vi "Open_File_for_write_check.vi"(8 "advisory dialog? (display:T)":bool=TRUE, 9 "append to file? (new file:F)":bool, 11 "file path":path) -> (0 "error out":errorcluster, 3 "refnum":refnum<file>)   [LabVIEW 2021]
doc: "Opens an existing file, creates a new file, or replaces an existing file, programmatically or interactively using dialog. You can optionally specify a dialog prompt, default file name, start path, or filter pattern, and you can specify open and deny modes when opening a file, plus group and permission when creating a new file. Use this VI with the intermediate Write File+ or Read File+ VIs described below.\n\nfile path is the path name of the file. If file path is empty (default value) or is Not A Path, the VI displays a File dialog box from which you can select a file. Error 43 occurs if the user cancels the dialog. \n\nfunction is the operation to perform:\n\n 0 (open) opens an existing file. Error 7 occurs if the file cannot be found.\n \n 1 (open or create) opens an existing file or creates a new file if one does not exist.\n\n 2 (create or replace) creates a new file or replaces a file if it exists and you give permission. Replacement is done by opening the file and setting EOF to 0. Error 43 occurs if the user elects to disallow the replacement using dialog. \n\n 3 (create) creates a new file. Error 8 occurs if the file already exists.\n\nadvisory dialog? Set TRUE (default) if you want a dialog if function=0 and the file does not exist, or if function=2 or 3 and the file exists.\n\nprompt is the message that appears below the list of files and directories in the file dialog.\n\ndefault name is the initial file name that appears in the selection box of the file dialog.\n\nstart path is the path name to the initially displayed directory in a file dialog. The default value is Not A Path, which is the path to the last directory shown in a file dialog.\n\npattern is the match pattern specification to display only certain types of files or directories. See the description of the File Dialog function for more information.\n\nerror in is a cluster of three elements (error?, code, and source) that describe the upstream error state, that is, the existance of any error preceeding the execution of the VI. The VI executes normally only if no incoming error exists; otherwise it merely passes the error in value to error out. error? is TRUE if an error occurred; the default value is FALSE. code is the error code; the default value is 0. source is in most cases the name of the VI or function that produced the error; the default value is an empty string.\n\nnew file path is the path of the file opened or created. You can use this output to determine the path of a file that you open or create using dialog. new file path returns Not A Path if the user selects Cancel from the dialog box.\n\nrefnum is the reference number of the open file. The value is Not A Refnum if the file cannot be opened.\n\nfile size is the size of the file in bytes; it is also the location of the end of file.\n\nerror out is a cluster of three elements (error?, code, and source) that describe the error state following the execution of the VI. If an incoming error does not exist, the VI executes normally and error out describes the VI's error state; if an incoming error exists, error out equals error in."
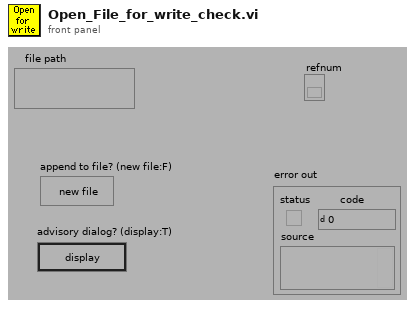
[diagram p1: front panel]
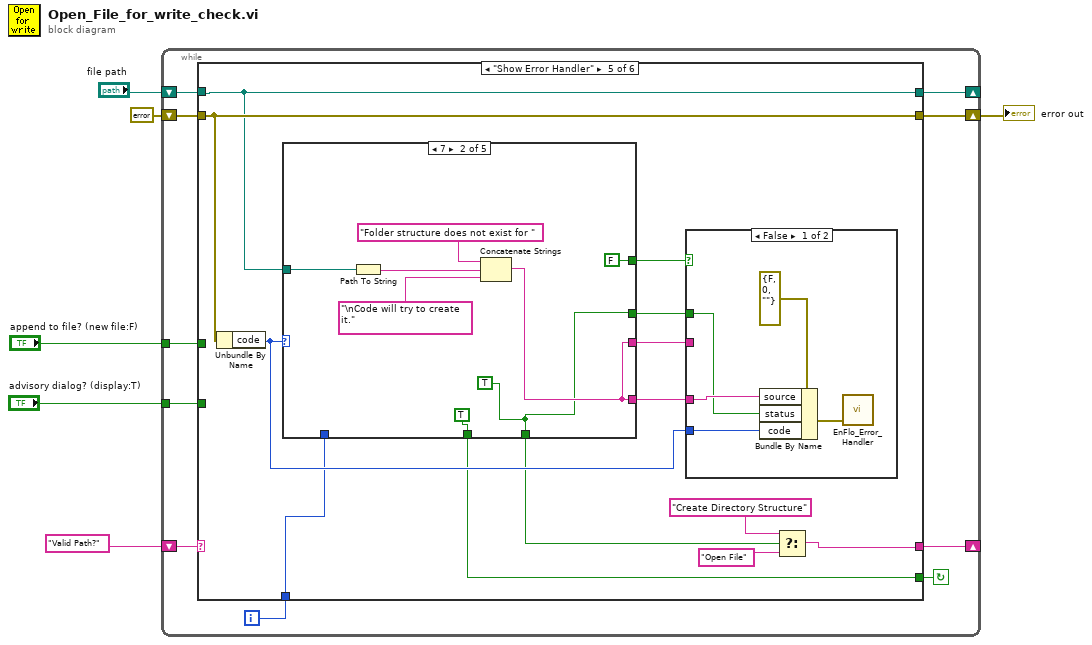
[diagram p0: block diagram]
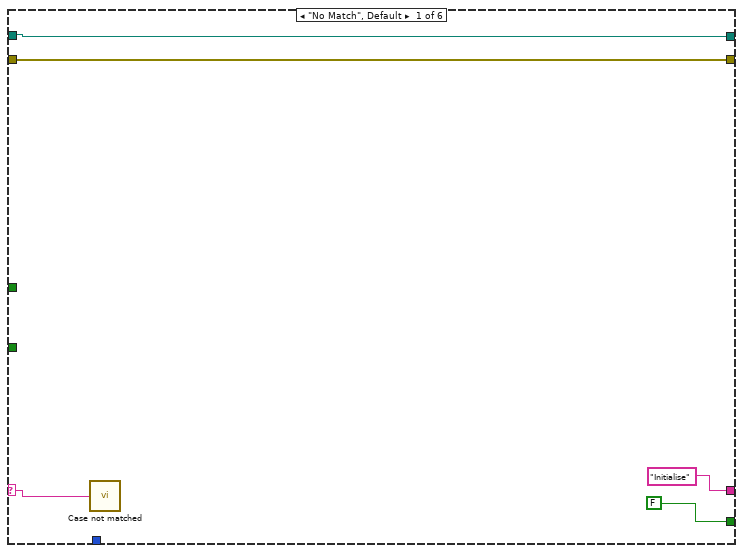
[diagram p2: hidden frame]
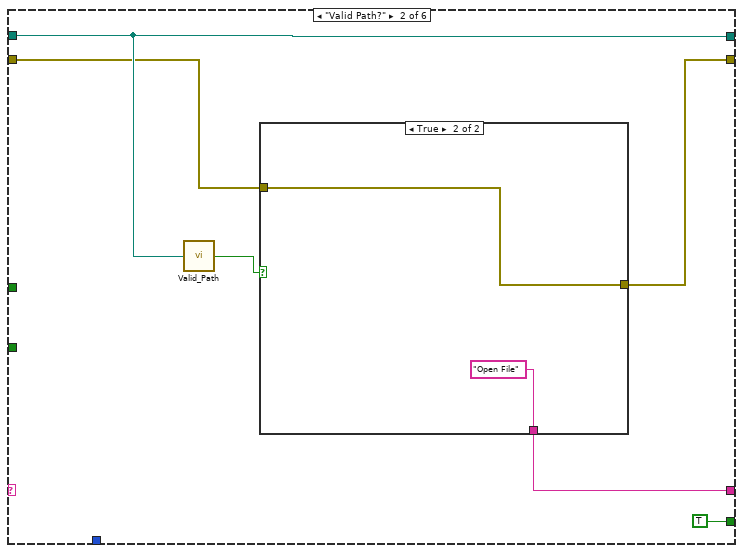
[diagram p3: hidden frame]
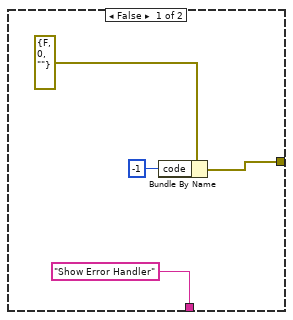
[diagram p4: hidden frame]
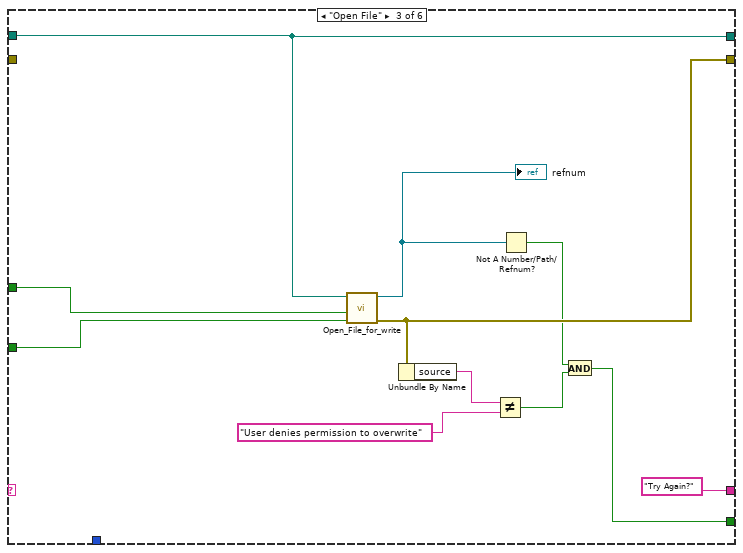
[diagram p5: hidden frame]
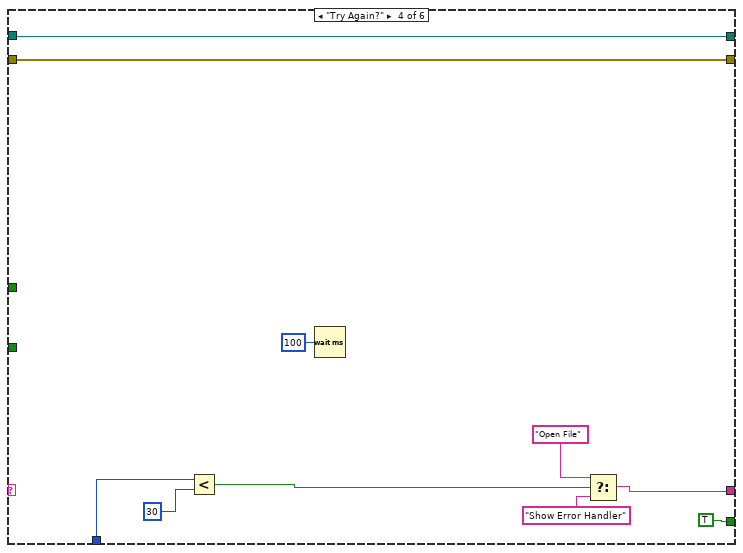
[diagram p6: hidden frame]
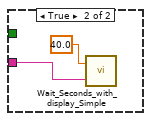
[diagram p7: hidden frame]
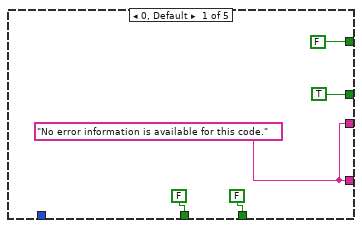
[diagram p8: hidden frame]
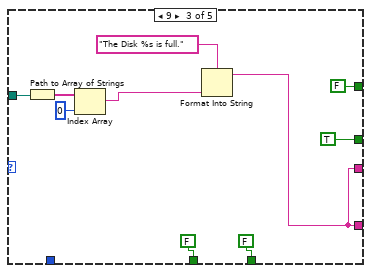
[diagram p9: hidden frame]
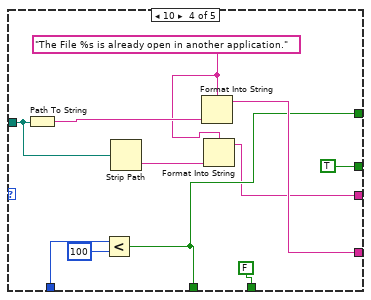
[diagram p10: hidden frame]
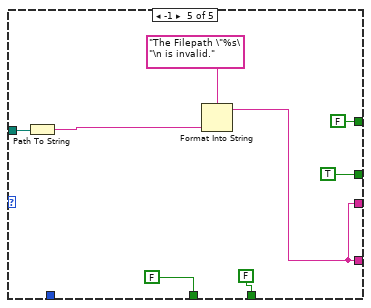
[diagram p11: hidden frame]
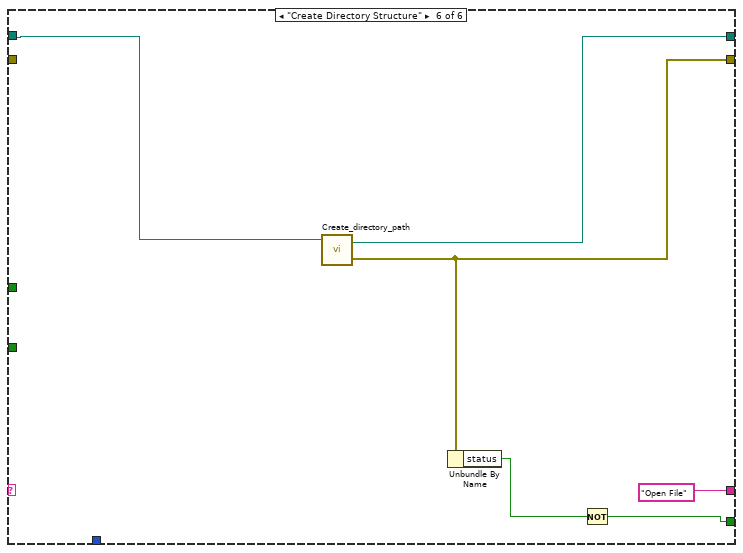
[diagram p12: hidden frame]
diagram:
  n1 = while {
    shift-left: "Valid Path?" -> [w14]
    shift-right: [w15] -> _
    tunnel: "append to file? (new file:F)" -> [w13]
    tunnel: "advisory dialog? (display:T)" -> [w12]
    shift-right: [w10] -> w3
    shift-left: errorcluster {"status"=FALSE, "code"=0, "source"=""} ("error out") -> [w7]
    shift-right: [w8] -> _
    shift-left: "file path" -> [w9]
    i -> [w11]
    stop <- w16 continue-if-true
    n2 = case shown="\"Show Error Handler\"" w14 {
      selector: w14 -> [w17 _ _ _ _ _]
      tunnel: [FALSE TRUE w34 TRUE w57 w119] -> w16
      tunnel: ["Initialise" w25 "Try Again?" w49 w67 "Open File"] -> w15
      tunnel: w13 -> [_ _ w43 _ _ _]
      tunnel: w12 -> [_ _ w42 _ _ _]
      tunnel: w9 -> [w19 w27 w40 w45 w63 w121]
      tunnel: w11 -> [_ _ _ w52 w58 _]
      tunnel: [w18 w23 w39 w46 w64 w117] -> w10
      tunnel: [w19 w27 w40 w45 w63 w122] -> w8
      tunnel: w7 -> [w18 w22 _ w46 w64 _]
      frame "No Match", Default {
        n3 = call "Case not matched.vi"("Case Name not Matched"=w17) -> ()
      }
      frame "Valid Path?" {
        n4 = call "Valid_Path.vi"("Filename"=w27) -> ("Valid Path?"=w26:bool)
        n5 = case shown="True" w26 {
          tunnel: ["Show Error Handler" "Open File"] -> w25
          tunnel: [w30 w32] -> w23
          tunnel: w22 -> [_ w32]
          frame False {
            n6 = Bundle By Name(cluster=errorcluster {"status"=FALSE, "code"=0, "source"=""} ("error in (no error)"), "code"=-1) -> (w30:errorcluster)
          }
          frame True {
          }
        }
      }
      frame "Open File" {
        n7 = call "Open_File_for_write.vi"("advisory dialog? (display:T)"=w42, "append to file? (new file:F)"=w43, "file path"=w40) -> ("error out"=w39:errorcluster, "refnum"=w41:refnum<file>)  [unwired: 7 out]
        "refnum" <- w41
        n8 = Unbundle By Name(w39) -> ("source"=w37:string)
        n9 = Not Equal?(x=w37, y="User denies permission to overwrite") -> (x != y?=w36:bool)
        n10 = Not A Number/Path/Refnum?(number/path/refnum=w41) -> (NaN/Path/Refnum?=w35:bool)
        n11 = And(x=w35, y=w36) -> (x .and. y?=w34:bool)
      }
      frame "Try Again?" {
        n12 = Less?(x=w52, y=30) -> (x < y?=w50:bool)
        n13 = Wait (ms)(milliseconds to wait=u32 100) -> ()  [unwired: 1 out]
        n14 = Select(t="Open File", s=w50, f="Show Error Handler") -> (s? t:f=w49:string)
      }
      frame "Show Error Handler" {
        n15 = Unbundle By Name(w64) -> ("code"=w61:i32)
        n16 = case shown="7" w61 {
          tunnel: w63 -> [_ w84 w97 w100 w116]
          tunnel: [w75 w81 w88 w108 w109] -> w62
          tunnel: [FALSE w80 FALSE FALSE FALSE] -> w60
          tunnel: [TRUE w80 TRUE TRUE TRUE] -> w59
          tunnel: [FALSE TRUE FALSE w102 FALSE] -> w57
          tunnel: w58 -> [_ _ _ w104 _]
          tunnel: [FALSE FALSE FALSE w102 FALSE] -> w56
          tunnel: [w75 w81 w88 w98 w109] -> w55
          frame 0, Default {
            w75 = "No error information is available for this code."
          }
          frame 7 {
            w80 = TRUE
            n17 = Path To String(path=w84) -> (string=w86:string)
            n18 = Concatenate Strings("Folder structure does not exist for ", w86, "\nCode will try to create it.") -> (w81:string)
          }
          frame 9 {
            n19 = Path to Array of Strings(0:w97) -> (2:w96:string[])  [unwired: 1 out]
            n20 = Index Array(array=w96, index=0 ("Index")) -> (element=w94:string)
            n21 = Format Into String(format string="The Disk %s is full." ("Format String"), w94) -> (resulting string=w88:string)  [unwired: 2 in, 1 out]
          }
          frame 10 {
            w101 = "The File %s is already open in another application." ("Format String")
            n22 = Path To String(path=w100) -> (string=w107:string)
            n23 = Less?(x=w104, y=100) -> (x < y?=w102:bool)
            n24 = Strip Path(path=w100) -> (name=w99:string)  [unwired: 1 out]
            n25 = Format Into String(format string=w101, w107) -> (resulting string=w108:string)  [unwired: 2 in, 1 out]
            n26 = Format Into String(format string=w101, w99) -> (resulting string=w98:string)  [unwired: 2 in, 1 out]
          }
          frame -1 {
            n27 = Path To String(path=w116) -> (string=w114:string)
            n28 = Format Into String(format string="The Filepath \"%s\"\n is invalid." ("Format String"), w114) -> (resulting string=w109:string)  [unwired: 2 in, 1 out]
          }
        }
        n29 = case shown="False" w56 {
          tunnel: w62 -> [w70 _]
          tunnel: w61 -> [w69 _]
          tunnel: w59 -> [w68 _]
          tunnel: w55 -> [_ w73]
          frame False {
            n30 = Bundle By Name(cluster=errorcluster {"status"=FALSE, "code"=0, "source"=""} ("error in (no error)"), "source"=w70, "status"=w68, "code"=w69) -> (w72:errorcluster)
            n31 = call "EnFlo_Error_Handler.vi"("error in (no error)"=w72) -> ()  [unwired: 2 in, 3 out]
          }
          frame True {
            n32 = call "Wait_Seconds_with_display_Simple.vi"("Message"=w73, "Seconds to wait"=40.0) -> ()  [unwired: 1 in, 1 out]
          }
        }
        n33 = Select(t="Create Directory Structure", s=w60, f="Open File") -> (s? t:f=w67:string)
      }
      frame "Create Directory Structure" {
        n34 = call "Create_directory_path.vi"("Path name"=w121) -> ("error out"=w117:errorcluster, "Path name Out"=w122:path)  [unwired: 2 in]
        n35 = Unbundle By Name(w117) -> ("status"=w118:bool)
        n36 = Not(x=w118) -> (.not. x?=w119:bool)
      }
    }
  }
  "error out" <- w3
